vi "Read Time.vi"(8 "error in (no error)":errorcluster, 11 "ControlDragSourceUpdateMsg In":refnum<class "ControlDragSourceUpdateMsg.lvclass">) -> (0 "error out":errorcluster, 2 "Time":u32, 3 "ControlDragSourceUpdateMsg Out":refnum<class "ControlDragSourceUpdateMsg.lvclass">)   [LabVIEW 2020, in "ActorEvents.lvlib" / "ControlDragSourceUpdateMsg.lvclass"]
uses:
  <vilib>/gpm_packages/@cs/mva-viewable/Source/ActorEvents/IEventAggregator Messages/ControlDragSourceUpdateMsg/ControlDragSourceUpdateMsg.lvclass
  <vilib>/gpm_packages/@cs/mva-viewable/Source/ActorEvents/IEventAggregator Messages/ControlDragSourceUpdateMsg/ControlDragSourceUpdateMsg.lvclass/ControlDragSourceUpdateMsg.ctl
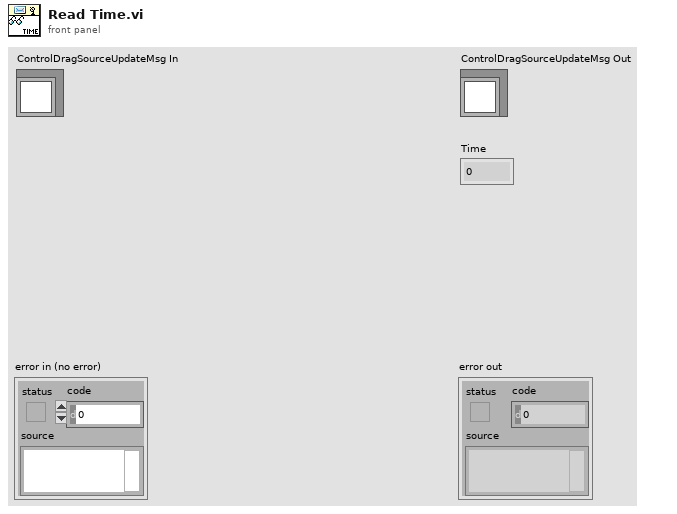
[diagram p1: front panel]
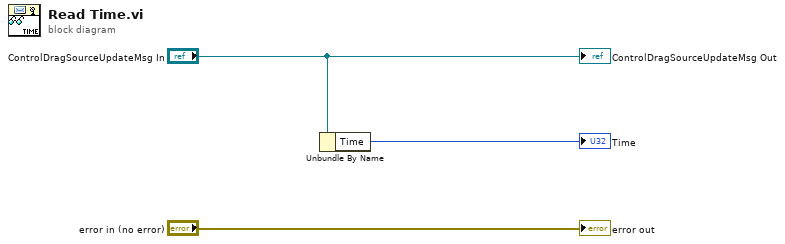
[diagram p0: block diagram]
diagram:
  n1 = Unbundle By Name("ControlDragSourceUpdateMsg In") -> ("Time"=→"Time":u32)
  "error out" <- "error in (no error)"
  "ControlDragSourceUpdateMsg Out" <- "ControlDragSourceUpdateMsg In"
